vi "DAQ EOL Station.vi"(3 "Reload Ok Refnum":refnum<vi>, 7 "ms":refnum<vi>, 9 "Exit Refnum":refnum<vi>, 10 "Restart Refnum":refnum<vi>, 11 "Part Type Refnum":refnum<vi>) -> ()   [LabVIEW 2018]
uses:
  type defs/EOL AI Channel Configuration Control.ctl
  <vilib>/Utility/error.llb/DialogType.ctl
  <vilib>/DAQmx/read.llb/DAQmx Read (Analog 2D DBL NChan NSamp).vi
  <vilib>/DAQmx/configure/timing.llb/DAQmx Timing (Sample Clock).vi
  <vilib>/DAQmx/miscellaneous.llb/DAQmx Fill In Error Info.vi
panel:
  out "Reload Config OK":bool
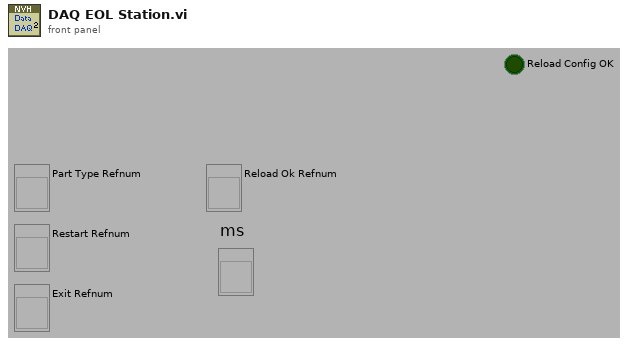
[diagram p1: front panel]
types:
  T1 = typedef "EOL AI Channel Configuration Control.ctl" = cluster{"input terminal configuration":i32, "minimum value":dbl, "maximum value":dbl, "physical channel":string, "channel name":string, "units":i32, "custom scale name":string, "type":enum16{"voltage", "thermocouple", "Amps"}}
  T2 = cluster{"millisecond timer value":u32, "AI Task ID":refnum<k21>, "Error":errorcluster, "Base Path":path, "AI Channels Configuration":T1[], "Part Type Refnum":refnum<vi>, "Reload Ok Refnum":refnum<vi>, "Restart Refnum":refnum<vi>, "Exit Refnum":refnum<vi>}
  T3 = enum16{"channel", "data files", "motion", "error table", "part config", "part setup", "tachometer"}
  T4 = enum16{"Initialize", "Read", "Write", "Read other"}
  T5 = typedef "DialogType.ctl" = u16
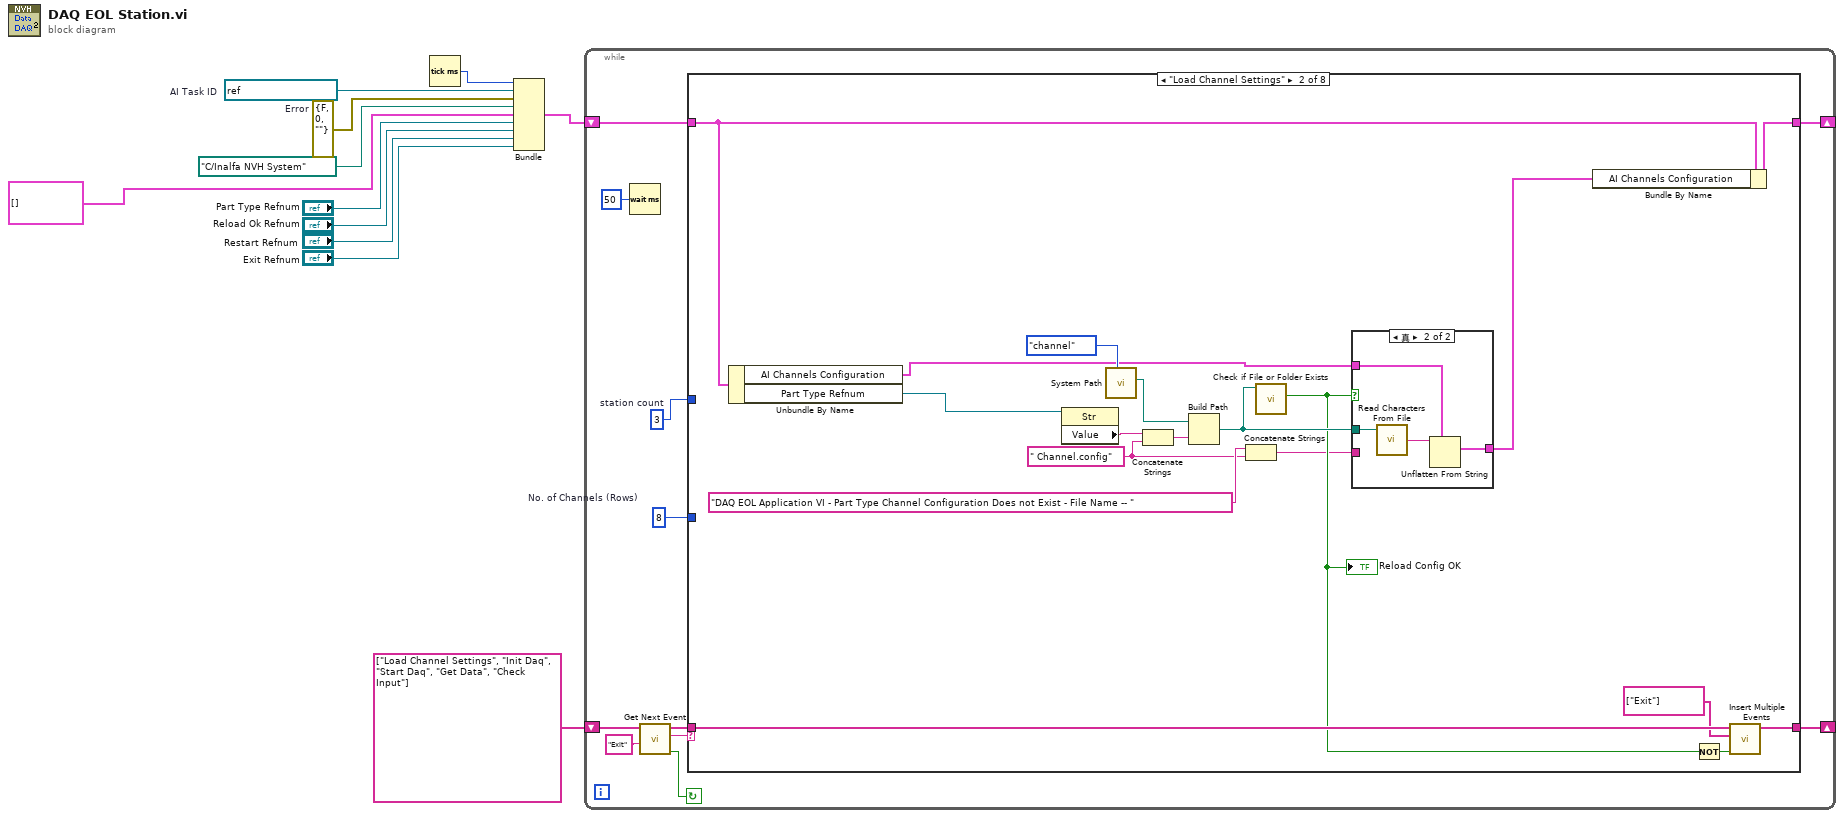
[diagram p0: block diagram]
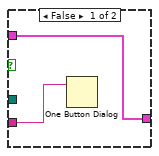
[diagram p3: hidden frame]
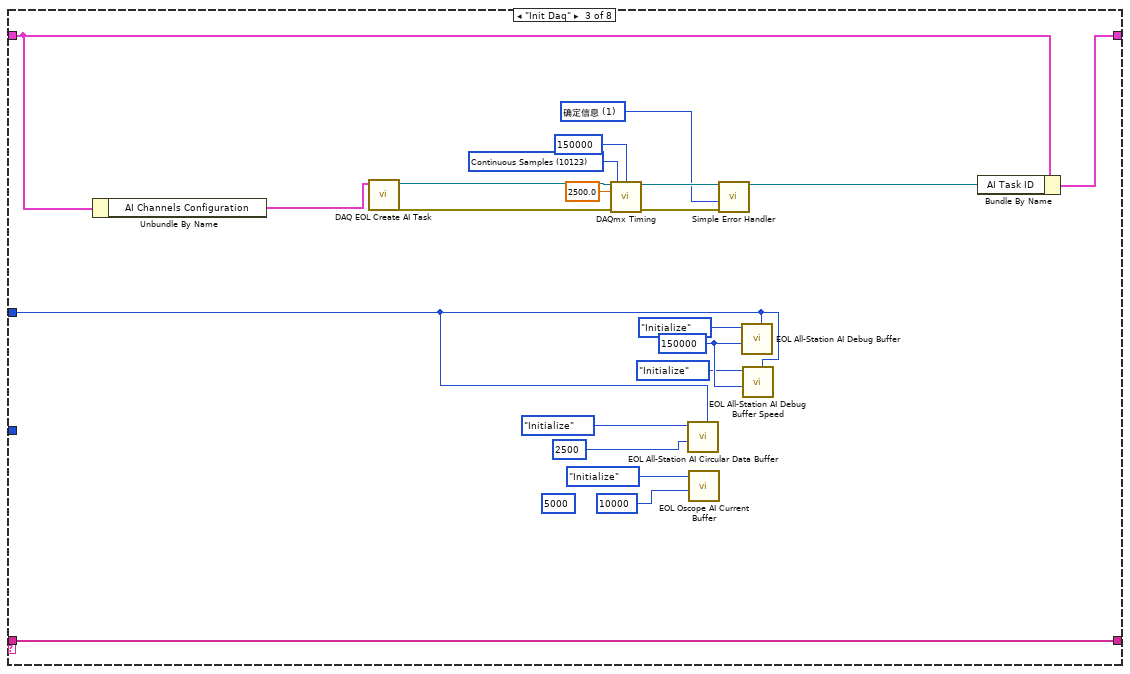
[diagram p4: hidden frame]
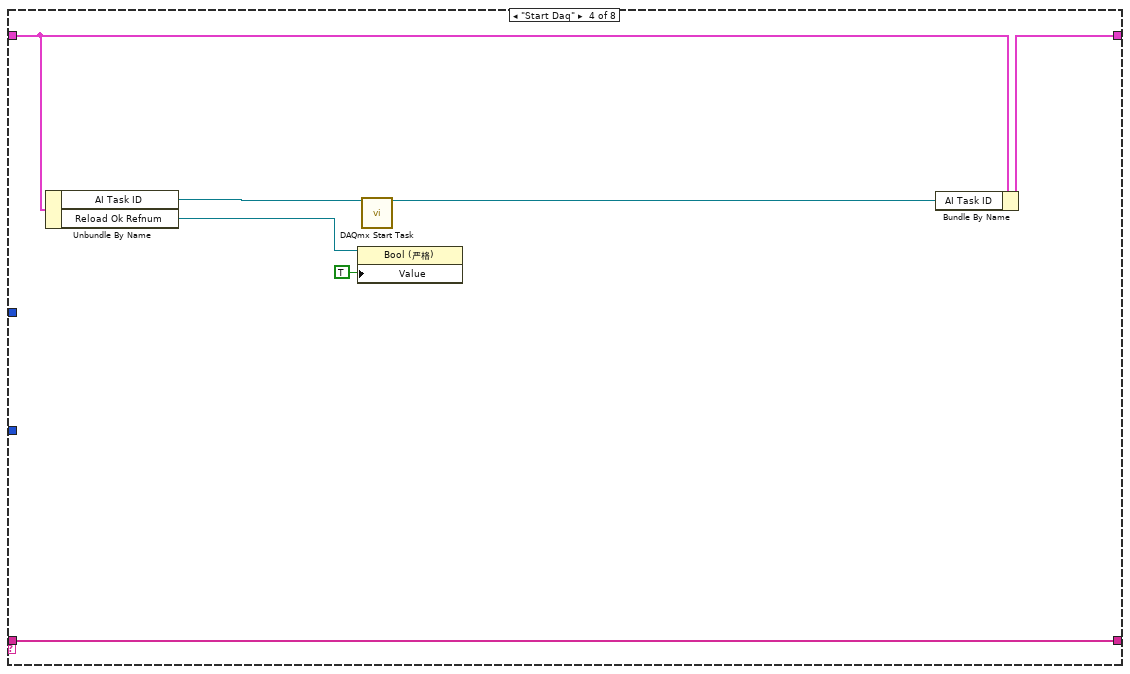
[diagram p5: hidden frame]
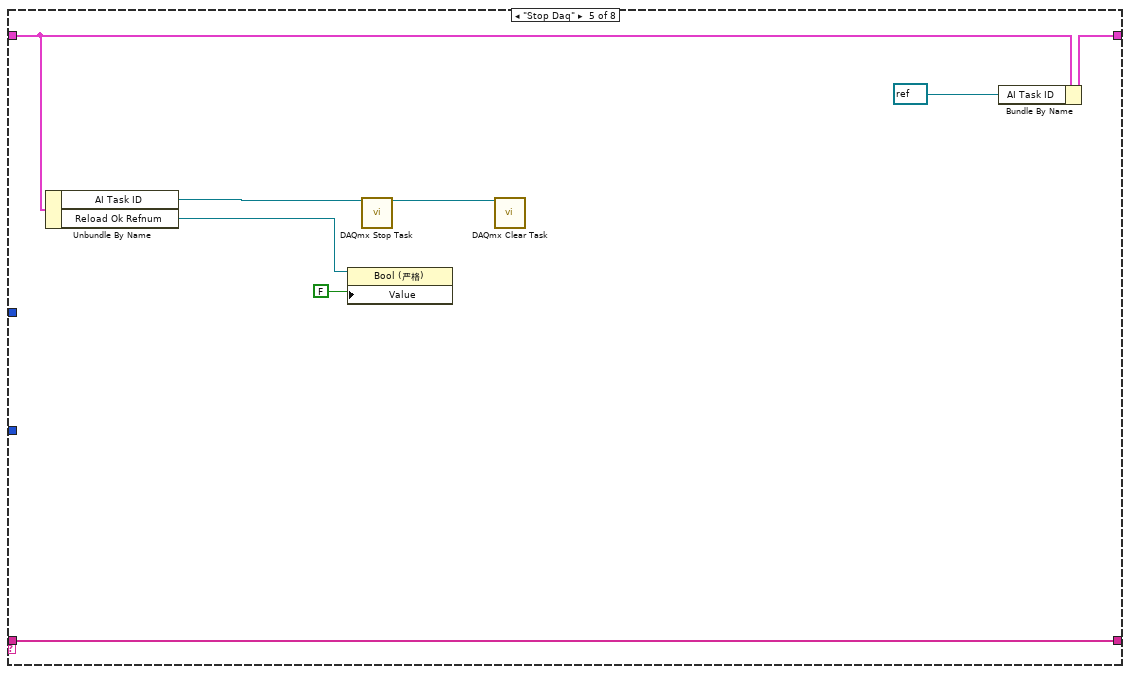
[diagram p6: hidden frame]
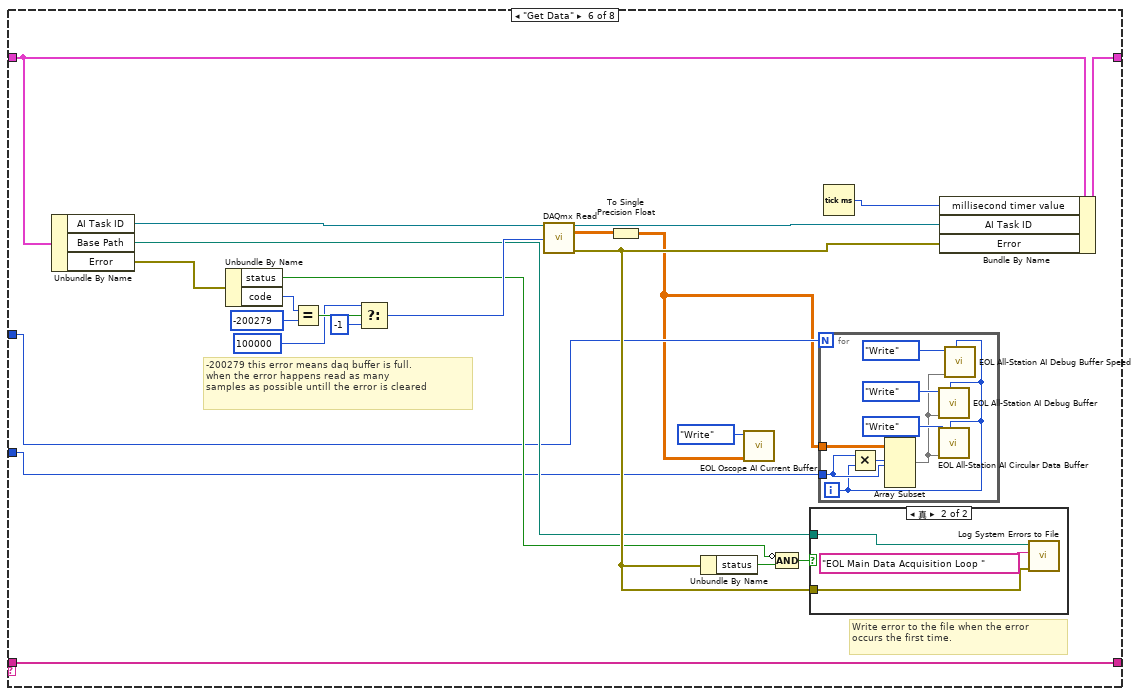
[diagram p7: hidden frame]
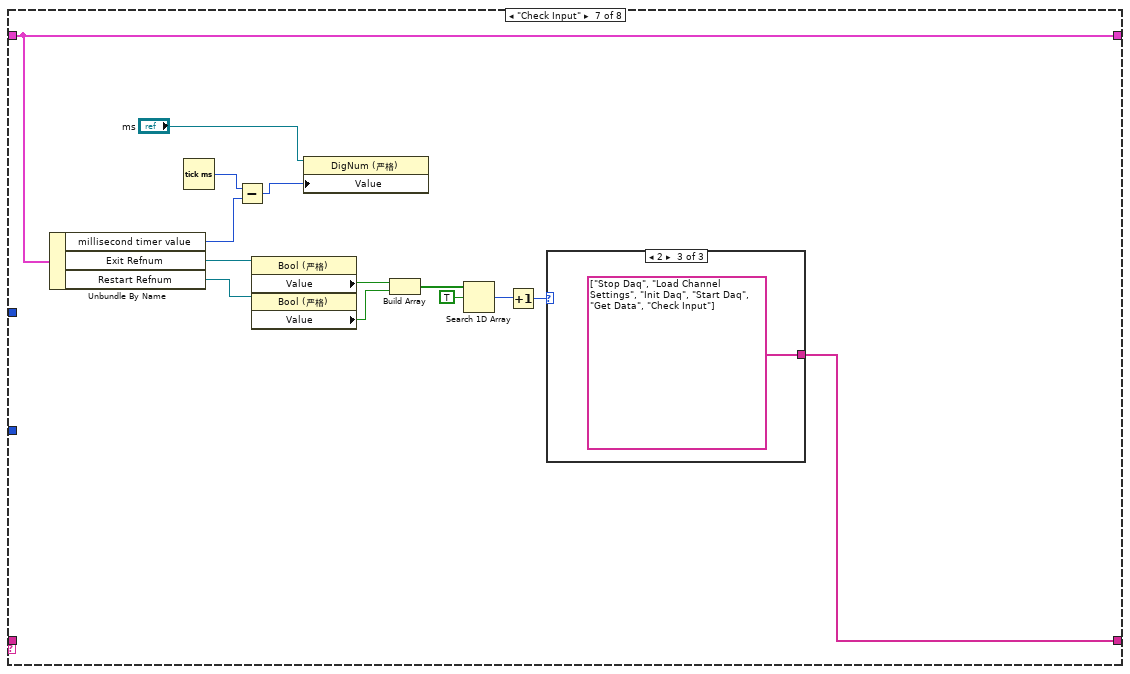
[diagram p9: hidden frame]
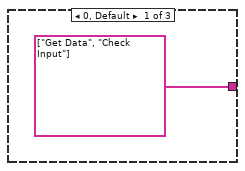
[diagram p10: hidden frame]
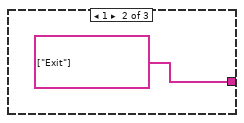
[diagram p11: hidden frame]
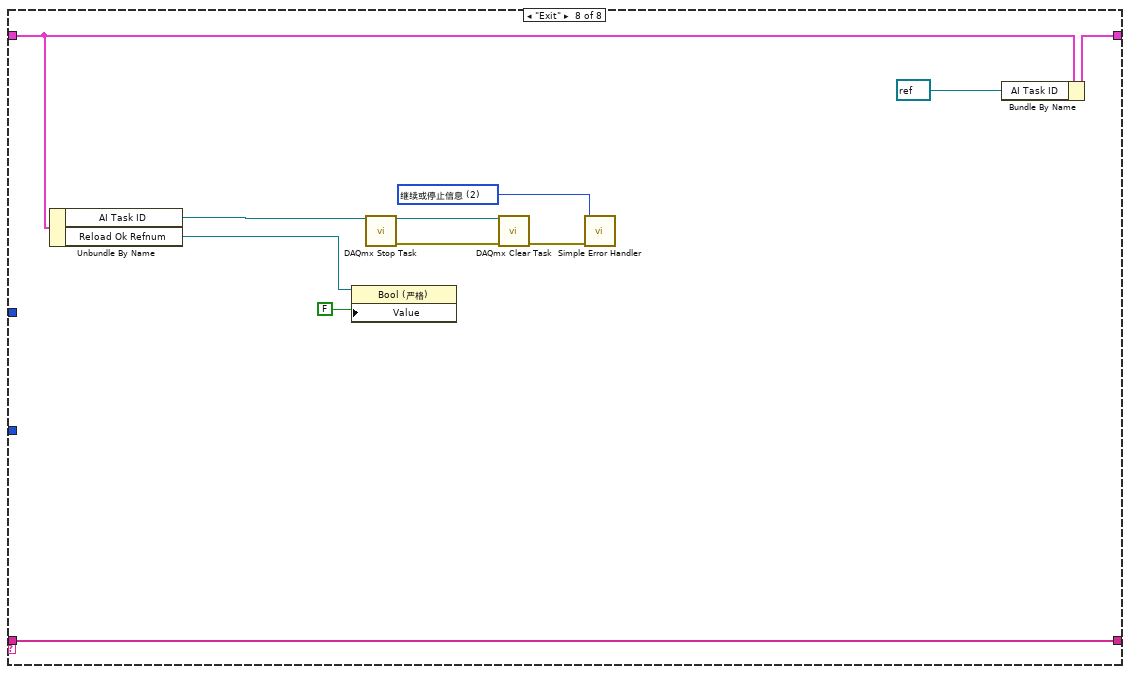
[diagram p12: hidden frame]
diagram:
  w10 = errorcluster {"status"=FALSE, "code"=0, "source"=""}  # Error
  w8 = refnum<k21> "NVH EOL DAQ"  # AI Task ID
  n1 = Tick Count (ms)() -> (millisecond timer value=w1:u32)
  n2 = Bundle("millisecond timer value"=w1, "AI Task ID"=w8, "Error"=w10, "Base Path"=path "C:/Inalfa NVH System", "AI Channels Configuration"=T1[] [], "Part Type Refnum"="Part Type Refnum", "Reload Ok Refnum"="Reload Ok Refnum", "Restart Refnum"="Restart Refnum", "Exit Refnum"="Exit Refnum") -> (w7:T2)  [unwired: 1 out]
  n3 = while {
    shift-right: [w19] -> _
    shift-left: string[] ["Load Channel Settings", "Init Daq", "Start Daq", "Get Data", "Check Input"] ("event queue out") -> [w18]
    shift-right: [w16] -> _
    shift-left: w7 -> [w17]
    stop <- w14 continue-if-true
    w12 = 8  # No. of Channels (Rows)
    w13 = 3  # station count
    n4 = Wait (ms)(milliseconds to wait=u32 50) -> ()  [unwired: 1 out]
    n5 = call "Get Next Event.vi"("Exit Event"="Exit", "event queue in"=w18) -> ("Condition (Exit:F)"=w14:bool, "next event"=w21:string, "event queue out"=w20:string[])  [unwired: 3 out]
    n6 = case shown="\"Load Channel Settings\"" w21 {
      tunnel: w20 -> [w24 w38 w68 w75 w83 w91 _ w145]
      tunnel: [w24 w37 w68 w75 w83 w91 w122 w145] -> w19
      tunnel: w17 -> [w23 w33 w61 w73 w77 w105 w131 w138]
      tunnel: [w23 w39 w64 w72 w76 w104 w131 w143] -> w16
      tunnel: w13 -> [_ _ w50 _ _ w87 _ _]
      tunnel: w12 -> [_ _ _ _ _ w88 _ _]
      frame "Error", Default {
      }
      frame "Load Channel Settings" {
        w28 = " Channel.config" ("string")
        n7 = Unbundle By Name(w33) -> ("AI Channels Configuration"=w25:T1[], "Part Type Refnum"=w32:refnum<vi>)
        n8 = property class="Str"(reference=w32) -> ("Value"=w34:string)  [unwired: 1 in, 2 out]
        n9 = call "System Path.vi"("file type"=T3."channel") -> ("new path"=w26:path)  [unwired: 9 in, 1 out]
        n10 = Concatenate Strings(w34, w28) -> (w40:string)
        n11 = Build Path(base path=w26, name or relative path=w40) -> (appended path=w41:path)
        n12 = Concatenate Strings("DAQ EOL Application VI - Part Type Channel Configuration Does not Exist - File Name -- " ("message"), w28) -> (w29:string)
        n13 = call <vilib>:"Check if File or Folder Exists.vi"("path"=w41) -> ("file or folder exists?"=w30:bool)  [unwired: 8 in, 2 out]
        "Reload Config OK" <- w30
        n14 = case shown="真" w30 {
          tunnel: w41 -> [_ w48]
          tunnel: [w44 w46] -> w31
          tunnel: w25 -> [w44 w45]
          tunnel: w29 -> [w43 _]
          frame False {
            n15 = One Button Dialog(message=w43) -> ()  [unwired: 1 in, 1 out]
          }
          frame True {
            n16 = call <vilib>:"Read Characters From File.vi"("file path (dialog if empty)"=w48) -> ("character string"=w47:string)  [unwired: 1 in, 7 out]
            n17 = Unflatten From String(type=w45, binary string=w47) -> (value=w46:T1[])  [unwired: 1 in, 4 out]
          }
        }
        n18 = Bundle By Name(cluster=w33, "AI Channels Configuration"=w31) -> (w39:T2)
        n19 = Not(x=w30) -> (.not. x?=w35:bool)
        n20 = call "Insert Multiple Events.vi"("Insert all? (T)"=w35, "Events to Insert"=string[] ["Exit"], "Event queue in"=w38) -> ("Event queue out"=w37:string[])  [unwired: 1 in, 3 out]
      }
      frame "Init Daq" {
        (unwired) 5000 ("Buffer Size (No. of Columns)")
        w52 = 150000 ("Buffer Size (seconds/2500)")
        w60 = T5 1 items=["无对话框", "确定信息", "继续或停止信息", "确定信息＋警告", "继续/停止+警告"] ("type of dialog (OK msg:1)")
        w67 = 10123 items=["Finite Samples"=10178, "Continuous Samples"=10123, "Hardware Timed Single Point"=12522] ("sample mode")
        n21 = Unbundle By Name(w61) -> ("AI Channels Configuration"=w49:T1[])
        n22 = call "DAQ EOL Create AI Task.vi"("AI Channel In"=w49) -> ("Error Out"=w59:errorcluster, "Analog Input Task"=w62:refnum<k21>)  [unwired: 1 in, 8 out]
        n23 = call-poly <vilib>:"DAQmx Timing.vi"("task/channels in"=w62, "sample mode"=w67, "samples per channel"=150000, "rate"=2500.0, "error in"=w59) -> ("task out"=w63:refnum<k21>, "error out"=w58:errorcluster)  [unwired: 2 in, 7 out]
        n24 = call "EOL All-Station AI Circular Data Buffer.vi"("number of stations"=w50, "Buffer Size (seconds/2500)"=2500 ("Buffer Size (No. of Columns)"), "Mode"=enum16{"Initialize", "Read", "Write"}."Initialize") -> ()  [unwired: 8 in, 1 out]
        n25 = call "EOL Oscope AI Current Buffer.vi"("Buffer Size (seconds/2500)"=10000 ("Buffer Size (No. of Columns)"), "Mode"=enum16{"Initialize", "Read", "Write"}."Initialize") -> ()  [unwired: 8 in, 2 out]
        n26 = call <vilib>:"Simple Error Handler.vi"("type of dialog (OK msg:1)"=w60, "error in (no error)"=w58) -> ()  [unwired: 3 in, 5 out]
        n27 = call "EOL All-Station AI Debug Buffer.vi"("number of stations"=w50, "Buffer Size (seconds/2500)"=w52, "Mode"=enum16{"Initialize", "Read", "Write"}."Initialize") -> ()  [unwired: 8 in, 1 out]
        n28 = call "EOL All-Station AI Debug Buffer Speed.vi"("number of stations"=w50, "Buffer Size (seconds/2500)"=w52, "Mode"=enum16{"Initialize", "Read", "Write"}."Initialize") -> ()  [unwired: 8 in, 1 out]
        n29 = Bundle By Name(cluster=w61, "AI Task ID"=w63) -> (w64:T2)
      }
      frame "Start Daq" {
        n30 = Unbundle By Name(w73) -> ("AI Task ID"=w74:refnum<k21>, "Reload Ok Refnum"=w70:refnum<vi>)
        n31 = property class="Bool (严格)"(reference=w70, "Value"=TRUE) -> ()  [unwired: 1 in, 2 out]
        n32 = call <vilib>:"DAQmx Start Task.vi"("task/channels in"=w74) -> ("task out"=w71:refnum<k21>)  [unwired: 1 in, 13 out]
        n33 = Bundle By Name(cluster=w73, "AI Task ID"=w71) -> (w72:T2)
      }
      frame "Stop Daq" {
        n34 = Unbundle By Name(w77) -> ("AI Task ID"=w82:refnum<k21>, "Reload Ok Refnum"=w80:refnum<vi>)
        n35 = property class="Bool (严格)"(reference=w80, "Value"=FALSE) -> ()  [unwired: 1 in, 2 out]
        n36 = call <vilib>:"DAQmx Stop Task.vi"("task/channels in"=w82) -> ("task out"=w81:refnum<k21>)  [unwired: 13 in, 1 out]
        n37 = call <vilib>:"DAQmx Clear Task.vi"("task in"=w81) -> ()  [unwired: 14 in, 1 out]
        n38 = Bundle By Name(cluster=w77, "AI Task ID"=refnum<k21> refnum ("task out")) -> (w76:T2)
      }
      frame "Get Data" {
        # "Write error to the file when the error\noccurs the first time."
        # "-200279 this error means daq buffer is full.\nwhen the error happens read as many \nsamples as possible untill the error is cleared"
        n39 = Unbundle By Name(w105) -> ("AI Task ID"=w106:refnum<k21>, "Base Path"=w92:path, "Error"=w97:errorcluster)
        n40 = Unbundle By Name(w97) -> ("status"=w90:bool, "code"=w98:i32)
        n41 = Equal?(x=w98, y=-200279 ("code 2")) -> (x = y?=w102:bool)
        n42 = Select(t=100000 ("number of samples per channel"), s=w102, f=-1) -> (s? t:f=w96:i32)
        n43 = call-poly <vilib>:"DAQmx Read.vi"("task/channels in"=w106, "number of samples per channel"=w96) -> ("task out"=w103:refnum<k21>, "data"=w89:dbl[][], "error out"=w93:errorcluster)  [unwired: 1 in, 10 out]
        n44 = To Single Precision Float(number=w89) -> (single precision float=w85:sgl[][])
        n45 = Unbundle By Name(w93) -> ("status"=w95:bool)
        n46 = call "EOL Oscope AI Current Buffer.vi"("Data to Write (Ch-Ro, Samp-Col)"=w85, "Mode"=T4."Write") -> ()  [unwired: 8 in, 2 out]
        n47 = Compound Arithmetic op=AND(invert w90, w95) -> (w94:bool)
        n48 = case shown="真" w94 {
          tunnel: w93 -> [_ w116]
          tunnel: w92 -> [_ w115]
          frame False {
          }
          frame True {
            n49 = call "Log System Errors to File.vi"("error out"=w116, "Comments"="EOL Main Data Acquisition Loop ", "Path"=w115) -> ()  [unwired: 9 out]
          }
        }
        n50 = for {
          N: w87 -> [_]
          tunnel: w85 -> [w114]
          tunnel: w88 -> [w112]
          i -> [w108]
          n51 = Multiply(x=w112, y=w108) -> (x*y=w113:i32)
          n52 = Array Subset(array=w114, index (row)=w113, length (row)=w112) -> (w107:sgl[][])  [unwired: 2 in]
          n53 = call "EOL All-Station AI Debug Buffer.vi"("station idx"=w108, "Data to Write (Ch-Ro, Samp-Col)"=w107, "Mode"=enum16{"Initialize", "Read", "Write"}."Write") -> ()  [unwired: 8 in, 1 out]
          n54 = call "EOL All-Station AI Circular Data Buffer.vi"("station idx"=w108, "Data to Write (Ch-Ro, Samp-Col)"=w107, "Mode"=enum16{"Initialize", "Read", "Write"}."Write") -> ()  [unwired: 8 in, 1 out]
          n55 = call "EOL All-Station AI Debug Buffer Speed.vi"("station idx"=w108, "Data to Write (Ch-Ro, Samp-Col)"=w107, "Mode"=enum16{"Initialize", "Read", "Write"}."Write") -> ()  [unwired: 8 in, 1 out]
        }
        n56 = Tick Count (ms)() -> (millisecond timer value=w84:u32)
        n57 = Bundle By Name(cluster=w105, "millisecond timer value"=w84, "AI Task ID"=w103, "Error"=w93) -> (w104:T2)
      }
      frame "Check Input" {
        n58 = Unbundle By Name(w131) -> ("millisecond timer value"=w120:u32, "Exit Refnum"=w130:refnum<vi>, "Restart Refnum"=w129:refnum<vi>)
        n59 = Tick Count (ms)() -> (millisecond timer value=w121:u32)
        n60 = Subtract(x=w121, y=w120) -> (x-y=w118:u32)
        n61 = property class="Bool (严格)"(reference=w130) -> ("Value"=w128:bool)  [unwired: 1 in, 2 out]
        n62 = property class="Bool (严格)"(reference=w129) -> ("Value"=w127:bool)  [unwired: 1 in, 2 out]
        n63 = property class="DigNum (严格)"(reference="ms", "Value"=w118) -> ()  [unwired: 1 in, 2 out]
        n64 = Build Array(w128, w127) -> (w126:bool[])
        n65 = Search 1D Array(1D array=w126, element=TRUE) -> (index of element=w124:i32)  [unwired: 1 in]
        n66 = Increment(x=w124) -> (x+1=w123:i32)
        n67 = case shown="2" w123 {
          tunnel: [string[] ["Get Data", "Check Input"] ("event queue out") string[] ["Exit"] ("event queue out") string[] ["Stop Daq", "Load Channel Settings", "Init Daq", "Start Daq", "Get Data", "Check Input"] ("event queue out")] -> w122
          frame 0, Default {
          }
          frame 1 {
          }
          frame 2 {
          }
        }
      }
      frame "Exit" {
        w135 = T5 2 items=["无对话框", "确定信息", "继续或停止信息", "确定信息＋警告", "继续/停止+警告"] ("type of dialog (OK msg:1)")
        n68 = Unbundle By Name(w138) -> ("AI Task ID"=w142:refnum<k21>, "Reload Ok Refnum"=w140:refnum<vi>)
        n69 = property class="Bool (严格)"(reference=w140, "Value"=FALSE) -> ()  [unwired: 1 in, 2 out]
        n70 = call <vilib>:"DAQmx Stop Task.vi"("task/channels in"=w142) -> ("task out"=w141:refnum<k21>, "error out"=w137:errorcluster)  [unwired: 13 in]
        n71 = call <vilib>:"DAQmx Clear Task.vi"("task in"=w141, "error in"=w137) -> ("error out"=w136:errorcluster)  [unwired: 13 in]
        n72 = call <vilib>:"Simple Error Handler.vi"("type of dialog (OK msg:1)"=w135, "error in (no error)"=w136) -> ()  [unwired: 3 in, 5 out]
        n73 = Bundle By Name(cluster=w138, "AI Task ID"=refnum<k21> refnum ("task out")) -> (w143:T2)
      }
    }
  }
